vi "Clean Up Panel.vi"(8 "error in (no error)":errorcluster, 9 "Conpane":refnum<vi>, 11 "VI Refnum":refnum<vi>) -> (0 "error out":errorcluster)   [LabVIEW 2020, in "Message Maker.lvlib"]
uses:
  Message Maker.lvlib
  <vilib>/Utility/miscctls.llb/LVPointTypeDef.ctl
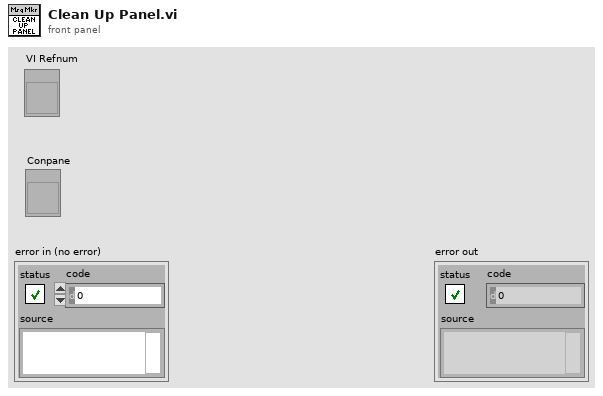
[diagram p1: front panel]
types:
  T1 = typedef "LVPointTypeDef.ctl" = cluster{"Horizontal":i16, "Vertical":i16}
  T2 = cluster{"Ctl Refnum":refnum<vi>, "width":i32, "height":i32}
  T3 = typedef "LVRectTypeDef.ctl" = cluster{"Left":i16, "Top":i16, "Right":i16, "Bottom":i16}
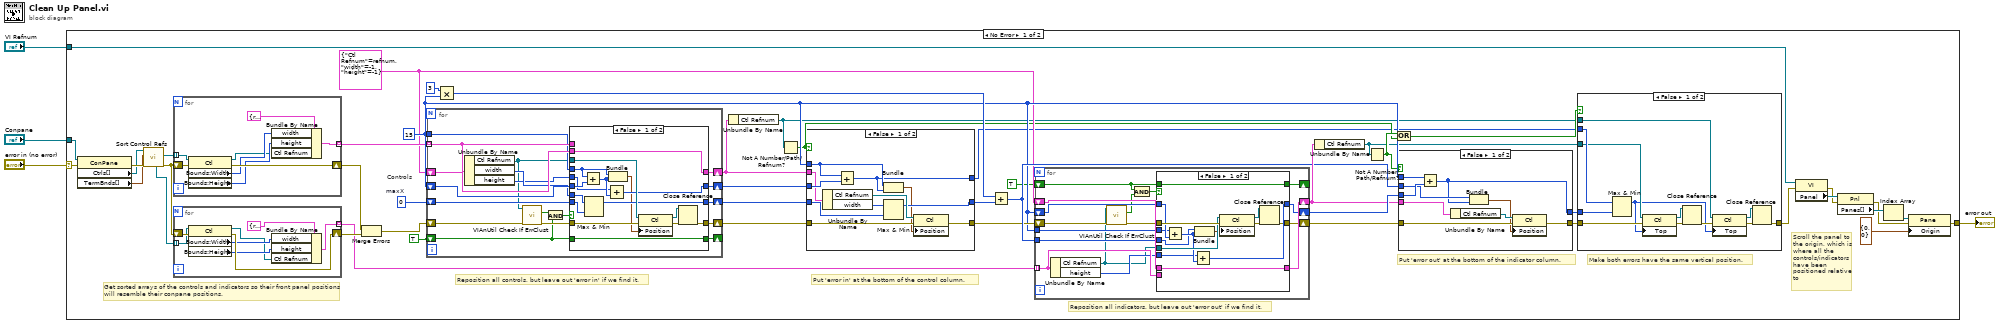
[diagram p0: block diagram]
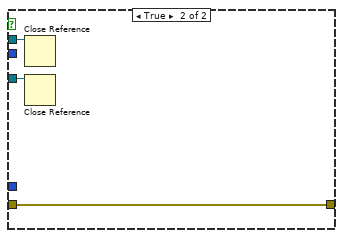
[diagram p2: hidden frame]
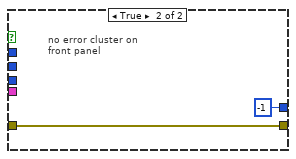
[diagram p3: hidden frame]
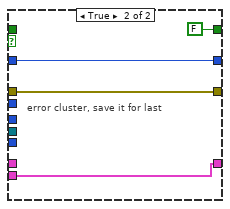
[diagram p4: hidden frame]
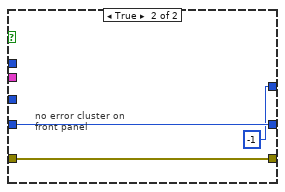
[diagram p5: hidden frame]
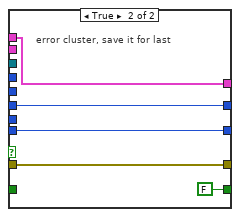
[diagram p6: hidden frame]
diagram:
  n1 = case shown="No Error" "error in (no error)" {
    selector: "error in (no error)" -> [w36 w181]
    tunnel: [w39 w181] -> w4
    tunnel: "VI Refnum" -> [w12 _]
    tunnel: "Conpane" -> [w32 _]
    frame No Error {
      w37 = 15 ("spacing")
      w23 = T2 {"Ctl Refnum"=refnum, "width"=-1, "height"=-1} ("control info prototype")
      w51 = 0  # maxX
      # "Scroll the panel to the origin, which is where all the controls/indicators have been positioned relative to"
      # "Make both errors have the same vertical position."
      # "Put 'error out' at the bottom of the indicator column."
      # "Reposition all indicators, but leave out 'error out' if we find it."
      # "Put 'error in' at the bottom of the control column."
      # "Reposition all controls, but leave out 'error in' if we find it."
      # "Get sorted arrays of the controls and indicators so their front panel positions will resemble their conpane positions."
      # "Controls"
      n2 = property class="ConPane"(reference=w32, error in=w36) -> (error out=w35:errorcluster, "Ctrls[]"=w34:refnum<vi>[], "TermBnds[]"=w33:T3[])  [unwired: 1 out]
      n3 = call "Sort Control Refs.vi"("error in (no error)"=w35, "Terminal Bounds[]"=w33, "Unsorted Refnums"=w34) -> ("error out"=w30:errorcluster, "Sorted Controls"=w31:refnum<vi>[], "Sorted Indicators"=w29:refnum<vi>[])  [unwired: 4 in, 2 out]
      n4 = for "Separate controls and indicators" {
        shift-right: [w179] -> w28
        shift-left: w30 -> [w180]
        tunnel: [w174] -> w25 mode=indexing
        tunnel: w31 -> [w173] mode=indexing
        n5 = property class="Ctl"(reference=w173, error in=w180) -> (reference out=w176:refnum<vi>, error out=w179:errorcluster, "Bounds:Width"=w178:u32, "Bounds:Height"=w177:u32)
        n6 = Bundle By Name(cluster=T2 {"Ctl Refnum"=refnum, "width"=0, "height"=0} ("control info prototype"), "width"=w178, "height"=w177, "Ctl Refnum"=w176) -> (w174:T2)
      }
      n7 = for "Separate controls and indicators" {
        shift-right: [w73] -> w27
        shift-left: w30 -> [w74]
        tunnel: [w68] -> w24 mode=indexing
        tunnel: w29 -> [w67] mode=indexing
        n8 = property class="Ctl"(reference=w67, error in=w74) -> (reference out=w70:refnum<vi>, error out=w73:errorcluster, "Bounds:Width"=w72:u32, "Bounds:Height"=w71:u32)
        n9 = Bundle By Name(cluster=T2 {"Ctl Refnum"=refnum, "width"=0, "height"=0} ("control info prototype"), "width"=w72, "height"=w71, "Ctl Refnum"=w70) -> (w68:T2)
      }
      n10 = Merge Errors(w28, w27) -> (w26:errorcluster)
      n11 = for "position controls" {
        shift-right: [w146] -> w49
        shift-left: w26 -> [w140]
        shift-right: [w148] -> w40
        shift-left: w23 -> [w149]
        tunnel: w25 -> [w147] mode=indexing
        shift-right: [w150] -> w48
        shift-left: w51 -> [w151]
        shift-right: [w144] -> w47
        shift-left: w37 -> [w145]
        tunnel: w37 -> [w141]
        shift-right: [w137] -> _
        shift-left: TRUE -> [w135]
        n12 = Unbundle By Name(w147) -> ("Ctl Refnum"=w138:refnum<vi>, "width"=w143:i32, "height"=w142:i32)
        n13 = call <vilib>:"VIAnUtil Check If ErrClust.vi"("error in (no error)"=w140, "Control in"=w138) -> ("error out"=w139:errorcluster, "Is error cluster?"=w136:bool)  [unwired: 7 in, 1 out]
        n14 = And(x=w136, y=w135) -> (x .and. y?=w134:bool)
        n15 = case shown="False" w134 {
          tunnel: w151 -> [w164 w172]
          tunnel: [w162 w172] -> w150
          tunnel: w149 -> [w167 _]
          tunnel: [w167 w171] -> w148
          tunnel: w147 -> [_ w171]
          tunnel: w139 -> [w166 w170]
          tunnel: [w156 w170] -> w146
          tunnel: w145 -> [w161 w169]
          tunnel: [w157 w169] -> w144
          tunnel: w143 -> [w163 _]
          tunnel: w142 -> [w158 _]
          tunnel: w138 -> [w165 _]
          tunnel: w141 -> [w160 _]
          tunnel: [w152 FALSE] -> w137
          tunnel: w135 -> [w152 _]
          frame False {
            n16 = Add(x=w160, y=w161) -> (x+y=w159:i32)
            n17 = Max & Min(x=w163, y=w164) -> (max(x,y)=w162:i32)  [unwired: 1 out]
            n18 = Add(x=w158, y=w159) -> (x+y=w157:i32)
            n19 = Bundle("spacing"=w160, w159) -> (w153:cluster{"spacing":i32, i32})  [unwired: 1 in]
            n20 = property class="Ctl"(reference=w165, error in=w166, "Position"=w153) -> (reference out=w154:refnum<vi>, error out=w155:errorcluster)
            n21 = Close Reference(reference=w154, error in (no error)=w155) -> (error out=w156:errorcluster)
          }
          frame True {
            # "error cluster, save it for last"
          }
        }
      }
      n22 = Multiply(x=3, y=w37) -> (x*y=w42:i32)
      n23 = Unbundle By Name(w40) -> ("Ctl Refnum"=w15:refnum<vi>)
      n24 = Not A Number/Path/Refnum?(number/path/refnum=w15) -> (NaN/Path/Refnum?=w21:bool)
      n25 = case "place error cluster last" shown="False" w21 {
        tunnel: w40 -> [w127 _]
        tunnel: w49 -> [w128 w132]
        tunnel: w48 -> [w129 w133]
        tunnel: w47 -> [w130 _]
        tunnel: [w123 w133] -> w46
        tunnel: [w120 w132] -> w38
        tunnel: w37 -> [w124 _]
        tunnel: [w121 -1] -> w17
        frame False {
          n26 = Unbundle By Name(w127) -> ("Ctl Refnum"=w126:refnum<vi>, "width"=w125:i32)
          n27 = Add(x=w124, y=w130) -> (x+y=w121:i32)
          n28 = Bundle("spacing"=w124, w121) -> (w122:cluster{"spacing":i32, i32})  [unwired: 1 in]
          n29 = Max & Min(x=w125, y=w129) -> (max(x,y)=w123:i32)  [unwired: 1 out]
          n30 = property class="Ctl"(reference=w126, error in=w128, "Position"=w122) -> (error out=w120:errorcluster)  [unwired: 1 out]
        }
        frame True {
          # "no error cluster on\nfront panel"
        }
      }
      n31 = Add(x=w42, y=w46) -> (x+y=w41:i32)
      n32 = for "position indicators" {
        shift-right: [w98] -> w44
        shift-left: w38 -> [w92]
        shift-right: [w100] -> w43
        shift-left: w23 -> [w101]
        tunnel: w24 -> [w99] mode=indexing
        shift-right: [w93] -> w45
        shift-left: w37 -> [w97]
        tunnel: w37 -> [w95]
        tunnel: w41 -> [w94]
        shift-right: [w89] -> _
        shift-left: TRUE -> [w87]
        n33 = Unbundle By Name(w99) -> ("Ctl Refnum"=w90:refnum<vi>, "height"=w96:i32)
        n34 = call <vilib>:"VIAnUtil Check If ErrClust.vi"("error in (no error)"=w92, "Control in"=w90) -> ("error out"=w91:errorcluster, "Is error cluster?"=w88:bool)  [unwired: 7 in, 1 out]
        n35 = And(x=w87, y=w88) -> (x .and. y?=w86:bool)
        n36 = case shown="False" w86 {
          tunnel: w94 -> [w107 _]
          tunnel: w101 -> [w115 _]
          tunnel: [w115 w119] -> w100
          tunnel: w99 -> [_ w119]
          tunnel: w91 -> [w114 w118]
          tunnel: [w104 w118] -> w98
          tunnel: w97 -> [w112 w117]
          tunnel: [w108 w117] -> w93
          tunnel: w96 -> [w109 _]
          tunnel: w90 -> [w113 _]
          tunnel: w95 -> [w111 _]
          tunnel: w87 -> [w102 _]
          tunnel: [w102 FALSE] -> w89
          frame False {
            n37 = Add(x=w111, y=w112) -> (x+y=w110:i32)
            n38 = Add(x=w109, y=w110) -> (x+y=w108:i32)
            n39 = Bundle(w107, w110) -> (w103:cluster{i32, i32})  [unwired: 1 in]
            n40 = property class="Ctl"(reference=w113, error in=w114, "Position"=w103) -> (reference out=w105:refnum<vi>, error out=w106:errorcluster)
            n41 = Close Reference(reference=w105, error in (no error)=w106) -> (error out=w104:errorcluster)
          }
          frame True {
            # "error cluster, save it for last"
          }
        }
      }
      n42 = Unbundle By Name(w43) -> ("Ctl Refnum"=w16:refnum<vi>)
      n43 = Not A Number/Path/Refnum?(number/path/refnum=w16) -> (NaN/Path/Refnum?=w22:bool)
      n44 = Or(x=w22, y=w21) -> (x .or. y?=w20:bool)
      n45 = case "place error cluster last" shown="False" w22 {
        tunnel: w43 -> [w81 _]
        tunnel: w44 -> [w82 w85]
        tunnel: w45 -> [w83 _]
        tunnel: [w75 w85] -> w19
        tunnel: w37 -> [w79 _]
        tunnel: w41 -> [w78 _]
        tunnel: [w76 -1] -> w18
        frame False {
          n46 = Add(x=w79, y=w83) -> (x+y=w76:i32)
          n47 = Unbundle By Name(w81) -> ("Ctl Refnum"=w80:refnum<vi>)
          n48 = Bundle(w78, w76) -> (w77:cluster{i32, i32})  [unwired: 1 in]
          n49 = property class="Ctl"(reference=w80, error in=w82, "Position"=w77) -> (error out=w75:errorcluster)  [unwired: 1 out]
        }
        frame True {
          # "no error cluster on\nfront panel"
        }
      }
      n50 = case shown="False" w20 {
        tunnel: w19 -> [w61 w66]
        tunnel: w18 -> [w62 _]
        tunnel: w17 -> [w63 _]
        tunnel: [w55 w66] -> w6
        tunnel: w16 -> [w60 w65]
        tunnel: w15 -> [w52 w64]
        frame False {
          n51 = Max & Min(x=w63, y=w62) -> (max(x,y)=w53:i32)  [unwired: 1 out]
          n52 = property class="Ctl"(reference=w60, error in=w61, "Top"=w53) -> (reference out=w58:refnum<vi>, error out=w59:errorcluster)
          n53 = Close Reference(reference=w58, error in (no error)=w59) -> (error out=w54:errorcluster)
          n54 = property class="Ctl"(reference=w52, error in=w54, "Top"=w53) -> (reference out=w57:refnum<vi>, error out=w56:errorcluster)
          n55 = Close Reference(reference=w57, error in (no error)=w56) -> (error out=w55:errorcluster)
        }
        frame True {
          n56 = Close Reference(reference=w64) -> ()  [unwired: 1 in, 1 out]
          n57 = Close Reference(reference=w65) -> ()  [unwired: 1 in, 1 out]
        }
      }
      n58 = property class="VI"(reference=w12, error in=w6) -> (error out=w7:errorcluster, "Panel"=w11:refnum<vi>)  [unwired: 1 out]
      n59 = property class="Pnl"(reference=w11, error in=w7) -> (error out=w5:errorcluster, "Panes[]"=w10:refnum<vi>[])  [unwired: 1 out]
      n60 = Index Array(array=w10) -> (element=w9:refnum<vi>)  [unwired: 1 in]
      n61 = property class="Pane"(reference=w9, error in=w5, "Origin"=T1 {"Horizontal"=0, "Vertical"=0}) -> (error out=w39:errorcluster)  [unwired: 1 out]
    }
    frame Error {
    }
  }
  "error out" <- w4
